vi "Remove Dependency.vi"(8 "error in (no error)":errorcluster, 10 "GUID":string, 11 "Attribute.Dependencies in":refnum<class "Attribute.Dependencies.lvclass">) -> (0 "error out":errorcluster, 3 "Attribute.Dependencies out":refnum<class "Attribute.Dependencies.lvclass">)   [LabVIEW 2021, in "smo.lvlib" / "Attribute.Dependencies.lvclass"]
uses:
  Attribute.Dependencies.lvclass
  Attribute.Dependencies.lvclass/Attribute.Dependencies.ctl
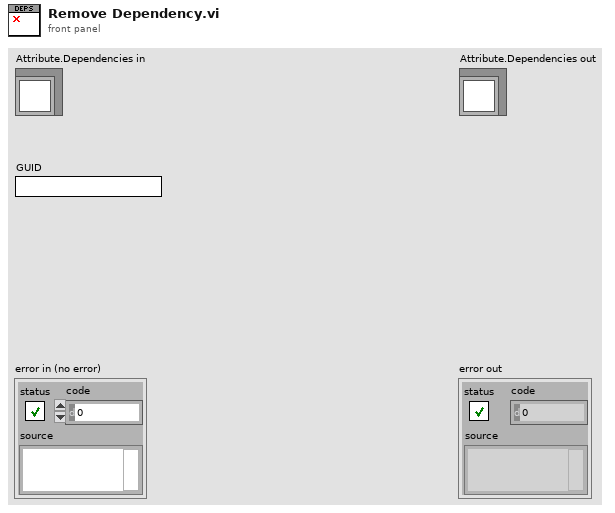
[diagram p1: front panel]
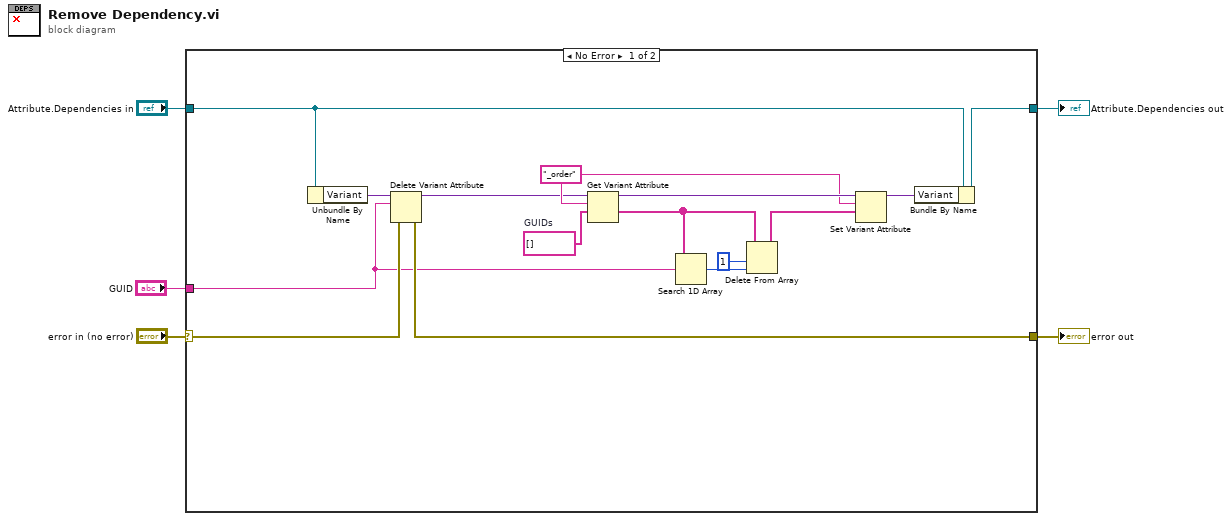
[diagram p0: block diagram]
diagram:
  n1 = case shown="No Error" "error in (no error)" {
    selector: "error in (no error)" -> [w17 w22]
    tunnel: [w16 w22] -> w4
    tunnel: [w20 w21] -> w2
    tunnel: "Attribute.Dependencies in" -> [w19 w21]
    tunnel: "GUID" -> [w10 _]
    frame No Error {
      w15 = string[] []  # GUIDs
      w13 = "_order" ("Attribute Name")
      n2 = Unbundle By Name(w19) -> ("Variant"=w18:variant)
      n3 = Delete Variant Attribute(4:w17, 6:w10, 7:w18) -> (0:w16:errorcluster, 3:w12:variant)  [unwired: 1 out]
      n4 = Get Variant Attribute(Variant=w12, name=w13, default value (empty Variant)=w15) -> (duplicate Variant=w14:variant, value=w9:string[])  [unwired: 1 in, 2 out]
      n5 = Search 1D Array(1D array=w9, element=w10) -> (index of element=w8:i32)  [unwired: 1 in]
      n6 = Delete From Array(array=w9, length=1, index=w8) -> (array with subset deleted=w6:string[])  [unwired: 1 out]
      n7 = Set Variant Attribute(Variant=w14, name=w13, value=w6) -> (Variant out=w11:variant)  [unwired: 1 in, 2 out]
      n8 = Bundle By Name(cluster=w19, "Variant"=w11) -> (w20:refnum<class "Attribute.Dependencies.lvclass">)
    }
    frame Error {
    }
  }
  "error out" <- w4
  "Attribute.Dependencies out" <- w2
